vi "dequeueForce.vi"(8 "error in (no error)":errorcluster) -> (0 "error out":errorcluster, 2 "Stop":bool, 3 "RawBits":u8[](array[numeric]))   [LabVIEW 2017, in "externalAquisition.lvlib"]
uses:
  externalAquisition.lvlib
  TypeDefs/QueueCommands.ctl
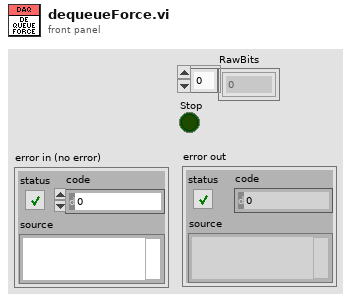
[diagram p1: front panel]
types:
  T1 = typedef "externalAquisition.lvlib/QueueCommands.ctl" = enum16{"get", "set"}
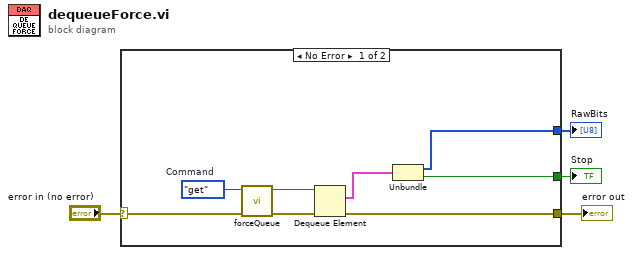
[diagram p0: block diagram]
diagram:
  n1 = case shown="No Error" "error in (no error)" {
    selector: "error in (no error)" -> [w12 w13]
    tunnel: [w5 w13] -> w3
    tunnel: [w7 _] -> w2
    tunnel: [w6 _] -> w1
    frame No Error {
      w11 = QueueCommands."get"  # Command
      n2 = call "forceQueue.vi"("error in (no error)"=w12, "Command"=w11) -> ("error out"=w10:errorcluster, "queue out"=w9:refnum<queue>)  [unwired: 8 in]
      n3 = Dequeue Element(queue=w9, error in (no error)=w10) -> (element=w8:cluster{u8[], "Stop":bool}, error out=w5:errorcluster)  [unwired: 1 in, 2 out]
      n4 = Unbundle(w8) -> (w7:u8[], "Stop"=w6:bool)
    }
    frame Error {
    }
  }
  "error out" <- w3
  "RawBits" <- w2
  "Stop" <- w1
